vi "Siargo Max Flow Rate Limit.vi"(8 "error in (no error)":errorcluster, 11 "Modbus API in":refnum<class "Modbus API.lvclass">) -> (0 "error out":errorcluster, 2 "MaxFlowRate":dbl, 3 "Modbus API out":refnum<class "Modbus API.lvclass">)   [LabVIEW 2020]
uses:
  <vilib>/NI/Modbus Library/API/Modbus API.lvclass
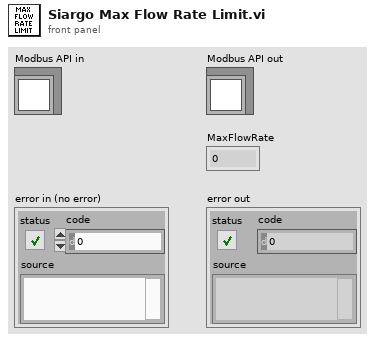
[diagram p1: front panel]
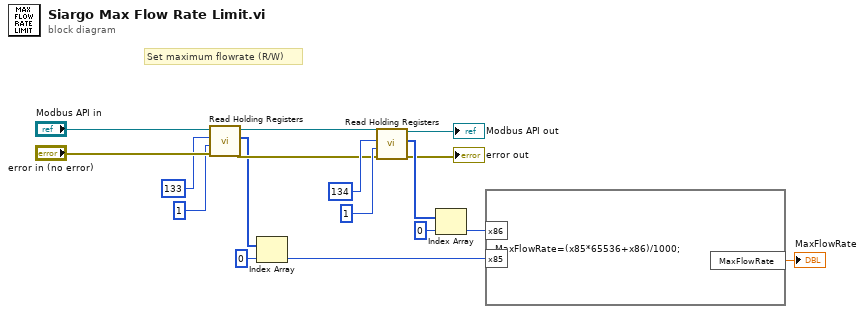
[diagram p0: block diagram]
diagram:
  # "Set maximum flowrate (R/W)"
  n1 = call-dynamic "Read Holding Registers.vi"("error in"="error in (no error)", "number of inputs"=u16 1, "starting address"=u16 133, "Modbus instance in"="Modbus API in") -> ("error out"=w10:errorcluster, "register values"=w9:u16[], "Modbus instance out"=w11:refnum<class "Modbus API.lvclass">)  [unwired: 5 in]
  n2 = Index Array(array=w9, index=0) -> (element=w5:u16)
  n3 = call-dynamic "Read Holding Registers.vi"("error in"=w10, "number of inputs"=u16 1, "starting address"=u16 134, "Modbus instance in"=w11) -> ("error out"=→"error out":errorcluster, "register values"=w8:u16[], "Modbus instance out"=→"Modbus API out":refnum<class "Modbus API.lvclass">)  [unwired: 5 in]
  n4 = Index Array(array=w8, index=0) -> (element=w4:u16)
  n5 = formula code="MaxFlowRate=(x85*65536+x86)/1000;"("x85"=w5, "x86"=w4) -> ("MaxFlowRate"=→"MaxFlowRate":dbl)
